vi "Connect.vi"(8 "error in (no error)":errorcluster, 10 "Connection String":string, 11 "SQLConnection Type":refnum<class "DBC.lvclass">) -> (0 "error out":errorcluster, 3 "SQLConnection out":refnum<class "DBC.lvclass">)   [LabVIEW 2020, in "ORM_DBC_Odbc.lvlib" / "DBC.lvclass"]
uses:
  DBC.lvclass
  C:/Program Files/National Instruments/LabVIEW 2020/vi.lib/Viviota/shared/ORM.lvlibp/ORM/DbConnection/DbConnection.lvclass
  System.Data
  <vilib>/Viviota/shared/ORM.lvlibp/ORM/DbConnection/Write connection.vi
  <vilib>/Viviota/shared/ORM.lvlibp/ORM/DbConnection/Write ColumnNameEqualsValueFormat.vi
  <vilib>/Viviota/shared/ORM.lvlibp/ORM/DbConnection/Write ColumnNameFormat.vi
  <vilib>/Viviota/shared/ORM.lvlibp/ORM/DbConnection/Write LastIdentityQuery.vi
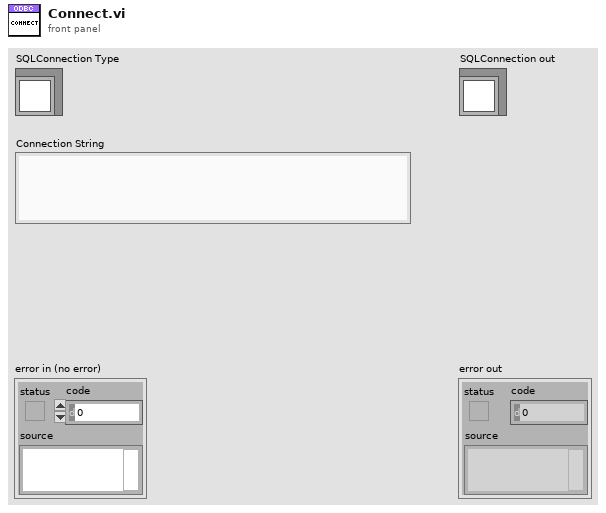
[diagram p1: front panel]
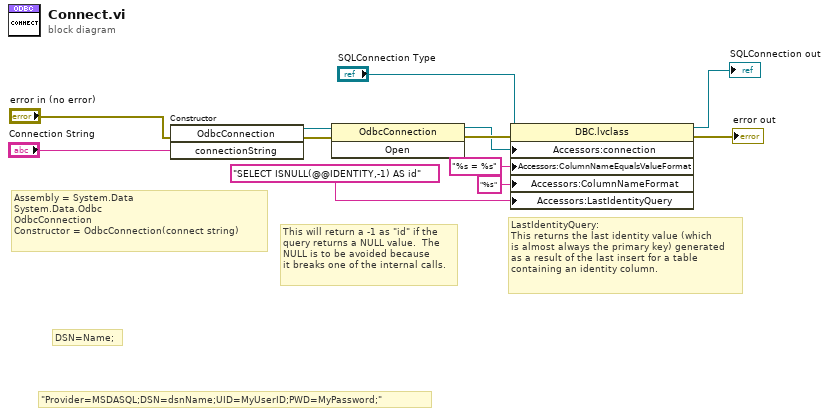
[diagram p0: block diagram]
diagram:
  # "\"Provider=MSDASQL;DSN=dsnName;UID=MyUserID;PWD=MyPassword;\""
  # "DSN=Name;"
  # "LastIdentityQuery:\nThis returns the last identity value (which\nis almost always the primary key) generated\nas a result of the last insert for a table \ncontaining an identity column."
  # "Assembly = System.Data\nSystem.Data.Odbc\nOdbcConnection\nConstructor = OdbcConnection(connect string)"
  # "This will return a -1 as \"id\" if the\nquery returns a NULL value.  The\nNULL is to be avoided because\nit breaks one of the internal calls."
  n1 = constructor class="OdbcConnection"(error in="error in (no error)", "connectionString"="Connection String") -> (reference out=w10:refnum<k24>, error out=w9:errorcluster)  [unwired: 2 in, 2 out]
  n2 = invoke class="OdbcConnection" method="Open"(reference=w10, error in=w9) -> (reference out=w6:refnum<k24>, error out=w7:errorcluster)  [unwired: 1 in, 1 out]
  n3 = property class="DBC.lvclass"(reference="SQLConnection Type", error in=w7, "Accessors:connection"=w6, "Accessors:ColumnNameEqualsValueFormat"="%s = %s" ("ColumnNameEqualsValueFormat"), "Accessors:ColumnNameFormat"="%s" ("ColumnNameFormat"), "Accessors:LastIdentityQuery"="SELECT ISNULL(@@IDENTITY,-1) AS id" ("LastIdentityQuery")) -> (reference out=→"SQLConnection out":refnum<class "DBC.lvclass">, error out=→"error out":errorcluster)
